vi "Get_AcquisitionBuffer.vi"(8 "error in":errorcluster, 11 "device handler in":u64) -> (0 "error out":errorcluster, 2 "AcquisitionBuffer":i8[](array[numeric]), 3 "device handler out":u64)   [LabVIEW 2014, in "PICam.lvlib"]
doc: "Picam_GetCameraID() returns the ID associates with a specified camera handle."
uses:
  PICam.lvlib
  Ctrls/PicamAcquisitionBufferWithFiller.ctl
  Picam32.dll
  Ctrls/PicamAcquisitionBufferWithoutFiller.ctl
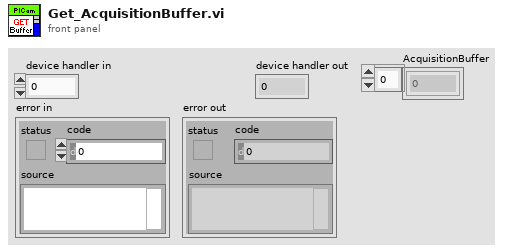
[diagram p1: front panel]
types:
  T1 = typedef "PICam.lvlib/PicamAcquisitionBufferWithFiller.ctl" = cluster{"memory":u32, "filler":u32, "memory size":u64}
  T2 = typedef "PICam.lvlib/PicamAcquisitionBufferWithoutFiller.ctl" = cluster{"memory":u64, "memory size":u64}
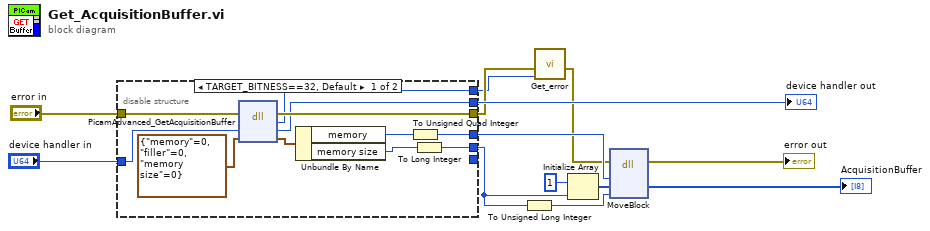
[diagram p0: block diagram]
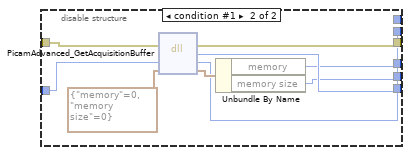
[diagram p2: hidden frame]
diagram:
  n1 = disable-structure shown="TARGET_BITNESS==32, Default" {
    disable-tunnel: [w22 w31] -> w3
    disable-tunnel: [_ w30] -> _
    disable-tunnel: [w21 w27] -> w11
    disable-tunnel: "error in" -> [w20 w32]
    disable-tunnel: "device handler in" -> [w19 w26]
    disable-tunnel: [w15 w29] -> w8
    disable-tunnel: [w16 w28] -> w7
    disable-tunnel: [w14 _] -> w1
    frame condition #0 (active) {
      n2 = dll-call lib="Picam32.dll" fn="PicamAdvanced_GetAcquisitionBuffer"(error in=w20, "camera_handle"=w19, "PicamAcquisitionBuffer"=T1 {"memory"=0, "filler"=0, "memory size"=0}) -> (error out=w22:errorcluster, "return type"=w14:i32, "camera_handle"=w21:u64, "PicamAcquisitionBuffer"=w24:T1)  [unwired: 2 in, 1 out]
      n3 = Unbundle By Name(w24) -> ("memory"=w17:u32, "memory size"=w18:u64)
      n4 = To Unsigned Quad Integer(1:w17) -> (0:w16:u64)
      n5 = To Long Integer(number=w18) -> (32bit integer=w15:i32)
    }
    frame condition #1 {
      n6 = dll-call lib="Picam32.dll" fn="PicamAdvanced_GetAcquisitionBuffer"(error in=w32, "camera_handle"=w26, "PicamAcquisitionBuffer"=T2 {"memory"=0, "memory size"=0}) -> (error out=w31:errorcluster, "return type"=w30:i32, "camera_handle"=w27:u64, "PicamAcquisitionBuffer"=w33:T2)  [unwired: 2 in, 1 out]
      n7 = Unbundle By Name(w33) -> ("memory"=w28:u64, "memory size"=w29:u64)
    }
  }
  "device handler out" <- w11
  n8 = To Unsigned Long Integer(number=w8) -> (unsigned 32bit integer=w4:u32)
  n9 = call "Get_error.vi"("PICam_Error"=w1, "error in (no error)"=w3) -> ("error out"=w2:errorcluster)  [unwired: 9 in]
  n10 = Initialize Array(1, w8) -> (w12:i32[])
  n11 = dll-call lib="LabVIEW" fn="MoveBlock"(error in=w2, "src"=w7, "dst"=w12, "size"=w4) -> (error out=→"error out":errorcluster, "dst"=→"AcquisitionBuffer":i32[])  [unwired: 5 in, 1 out]
